vi "TangoAttributeAttributeDataReadyEventTest.vi"() -> ()   [LabVIEW 2013, in "examples.lvlib"]
uses:
  examples.lvlib
  vis/lv-2013/tango_vi.llb/tango.lvlib
panel:
  in  "DRE attribute name":string
  out "attribute data ready":T1
  out "?":string="\n1. Device Name: the name of a Tango device having (at least) a \"data ready enabled\" attribute\n\n2. DRE attribute name: the name of a \"data ready enabled attribute\" \n\n3. Start the Vi\n\n4. The data counter of the data ready cluster should be incremented each time a data ready event is received"
  in  "?":bool
  in  "Device Name":string
  # "TANGO \"ATTRIBUTE DATA READY\" EVENT DEMO"
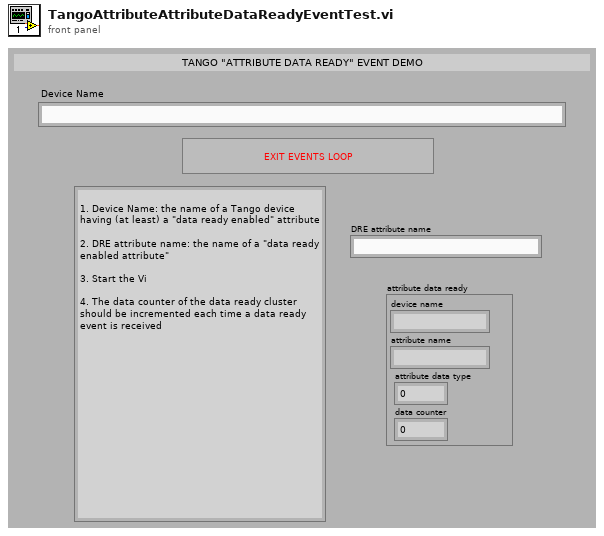
[diagram p1: front panel]
types:
  T1 = cluster{"device name":string, "attribute name":string, "attribute data type":i16, "data counter":i16}
  T2 = cluster{"user event ref":refnum<user-event>, "user event reg refnum":refnum<event-registration>}
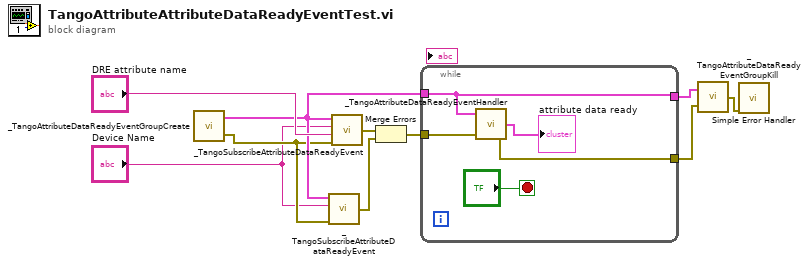
[diagram p0: block diagram]
diagram:
  n1 = call "_TangoAttributeDataReadyEventGroupCreate.vi"() -> ("attribute data ready event ref"=w8:T2, "error out"=w7:errorcluster)  [unwired: 1 in]
  n2 = call "_TangoSubscribeAttributeDataReadyEvent.vi"("error in"=w7, "device name"="Device Name", "attribute data ready event ref"=w8) -> ("error out"=w5:errorcluster)  [unwired: 1 in]
  n3 = call "_TangoSubscribeAttributeDataReadyEvent.vi"("error in"=w7, "attribute name"="DRE attribute name", "device name"="Device Name", "attribute data ready event ref"=w8) -> ("error out"=w6:errorcluster)
  n4 = Merge Errors(w6, w5) -> (w4:errorcluster)
  n5 = while {
    tunnel: w8 -> [w14]
    tunnel: w4 -> [w15]
    tunnel: [w14] -> w9
    tunnel: [w11] -> w2
    stop <- "?" stop-if-true
    n6 = call "_TangoAttributeDataReadyEventHandler.vi"("error in"=w15, "attribute data ready event ref"=w14) -> ("error out"=w11:errorcluster, "attribute data ready"=→"attribute data ready":T1)  [unwired: 1 in, 1 out]
  }
  n7 = call "_TangoAttributeDataReadyEventGroupKill.vi"("error in"=w2, "attribute data ready event ref"=w9) -> ("error out"=w1:errorcluster)
  n8 = call <vilib>:"Simple Error Handler.vi"("error in (no error)"=w1) -> ()  [unwired: 4 in, 5 out]
